vi "RelayToggle.vi"(8 "error in":errorcluster, 10 "Power":bool, 11 "Relay":T1) -> (0 "error out":errorcluster)   [LabVIEW 2017]
uses:
  Type Defs/Relays.ctl
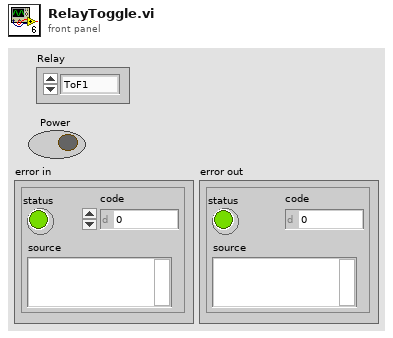
[diagram p1: front panel]
types:
  T1 = typedef "Relays.ctl" = enum16{"ToF1", "ToF2", "ToF3", "ToF4", "ToF5", "ToF6", "ToF7", "ToF8", "SensePwr", "All"}
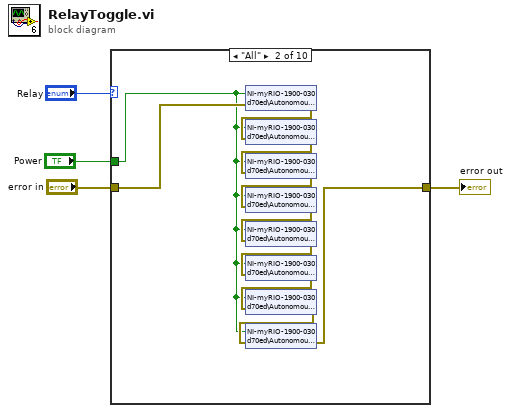
[diagram p0: block diagram]
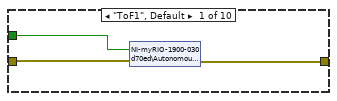
[diagram p2: hidden frame]
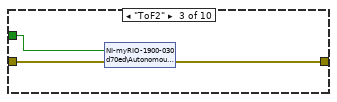
[diagram p3: hidden frame]
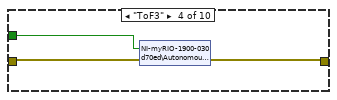
[diagram p4: hidden frame]
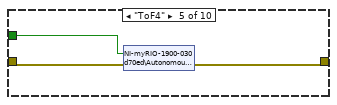
[diagram p5: hidden frame]
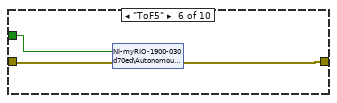
[diagram p6: hidden frame]
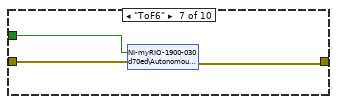
[diagram p7: hidden frame]
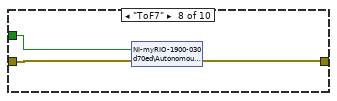
[diagram p8: hidden frame]
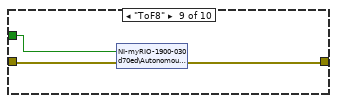
[diagram p9: hidden frame]
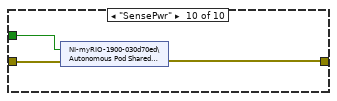
[diagram p10: hidden frame]
diagram:
  n1 = case shown="\"All\"" "Relay" {
    tunnel: [w5 w8 w18 w21 w24 w27 w30 w33 w36 w40] -> w2
    tunnel: "error in" -> [w6 w10 w20 w23 w26 w29 w32 w35 w38 w41]
    tunnel: "Power" -> [w7 w9 w19 w22 w25 w28 w31 w34 w37 w39]
    frame "ToF1", Default {
      n2 = shared-variable "NI-myRIO-1900-030d70ed\\Autonomous Pod Shared Variables.lvlib\\ToF1"(w7, error in=w6) -> (error out=w5:errorcluster)
    }
    frame "All" {
      n3 = shared-variable "NI-myRIO-1900-030d70ed\\Autonomous Pod Shared Variables.lvlib\\ToF1"(w9, error in=w10) -> (error out=w11:errorcluster)
      n4 = shared-variable "NI-myRIO-1900-030d70ed\\Autonomous Pod Shared Variables.lvlib\\ToF2"(w9, error in=w11) -> (error out=w12:errorcluster)
      n5 = shared-variable "NI-myRIO-1900-030d70ed\\Autonomous Pod Shared Variables.lvlib\\ToF3"(w9, error in=w12) -> (error out=w13:errorcluster)
      n6 = shared-variable "NI-myRIO-1900-030d70ed\\Autonomous Pod Shared Variables.lvlib\\ToF4"(w9, error in=w13) -> (error out=w14:errorcluster)
      n7 = shared-variable "NI-myRIO-1900-030d70ed\\Autonomous Pod Shared Variables.lvlib\\ToF5"(w9, error in=w14) -> (error out=w15:errorcluster)
      n8 = shared-variable "NI-myRIO-1900-030d70ed\\Autonomous Pod Shared Variables.lvlib\\ToF6"(w9, error in=w15) -> (error out=w16:errorcluster)
      n9 = shared-variable "NI-myRIO-1900-030d70ed\\Autonomous Pod Shared Variables.lvlib\\ToF7"(w9, error in=w16) -> (error out=w17:errorcluster)
      n10 = shared-variable "NI-myRIO-1900-030d70ed\\Autonomous Pod Shared Variables.lvlib\\ToF8"(w9, error in=w17) -> (error out=w8:errorcluster)
    }
    frame "ToF2" {
      n11 = shared-variable "NI-myRIO-1900-030d70ed\\Autonomous Pod Shared Variables.lvlib\\ToF2"(w19, error in=w20) -> (error out=w18:errorcluster)
    }
    frame "ToF3" {
      n12 = shared-variable "NI-myRIO-1900-030d70ed\\Autonomous Pod Shared Variables.lvlib\\ToF3"(w22, error in=w23) -> (error out=w21:errorcluster)
    }
    frame "ToF4" {
      n13 = shared-variable "NI-myRIO-1900-030d70ed\\Autonomous Pod Shared Variables.lvlib\\ToF4"(w25, error in=w26) -> (error out=w24:errorcluster)
    }
    frame "ToF5" {
      n14 = shared-variable "NI-myRIO-1900-030d70ed\\Autonomous Pod Shared Variables.lvlib\\ToF5"(w28, error in=w29) -> (error out=w27:errorcluster)
    }
    frame "ToF6" {
      n15 = shared-variable "NI-myRIO-1900-030d70ed\\Autonomous Pod Shared Variables.lvlib\\ToF6"(w31, error in=w32) -> (error out=w30:errorcluster)
    }
    frame "ToF7" {
      n16 = shared-variable "NI-myRIO-1900-030d70ed\\Autonomous Pod Shared Variables.lvlib\\ToF7"(w34, error in=w35) -> (error out=w33:errorcluster)
    }
    frame "ToF8" {
      n17 = shared-variable "NI-myRIO-1900-030d70ed\\Autonomous Pod Shared Variables.lvlib\\ToF8"(w37, error in=w38) -> (error out=w36:errorcluster)
    }
    frame "SensePwr" {
      n18 = shared-variable "NI-myRIO-1900-030d70ed\\Autonomous Pod Shared Variables.lvlib\\SensePower"(w39, error in=w41) -> (error out=w40:errorcluster)
    }
  }
  "error out" <- w2
